vi "timeout determiner.vi"(11 "Status":T1={"VI"={"error"={"status"=FALSE, "code"=0, "source"=""}, "isExiting?"=FALSE}, "UserLoggedIn?"=FALSE, "AVI Refnum"=refnum, "video path"=path "", "Frame Data"={"Width"=0, "Height"=0, "Frames Per Second"=0, "Codec"="", "Has Data"=FALSE}, "Number of Frames"=0, "Frame Number"=0, "Image Placeholder"=refnum, "Image Output"=refnum, "First Frame?"=TRUE, "Running?"=FALSE, "ROI Type"=enum."Line ROI", "ROI Descriptor"={"Global Rectangle"=[], "Contours"=[]}, "ROI Present?"=FALSE, "Filter Set?"=FALSE, "Loop?"=FALSE, "Filtering?"=FALSE, "Filter Parameters"={"Sigma"=1.0, "HThresh"=0.7, "LThres"=0.2, "WindowSize"=9}} {"Filter Parameters"."LThres" min=0 max=1 format="%.2f"; "Filter Parameters"."HThresh" min=0 max=1 format="%.2f"; "Filter Parameters"."Sigma" min=0 max=1 format="%.2f"; "ROI Descriptor"."Contours"."Type" items=["No Selection", "Point", "Line", "Rectangle", "Oval", "Polygon", "Freehand Region", "Annulus", "Unused2", "Unused3", "Broken Line", "Freehand Line", "Rotated Rectangle"]}) -> (3 "Numeric":i32)   [LabVIEW 2018]
uses:
  Status.ctl
  <vilib>/vision/Avi.llb/IMAQ AVI2 Refnum.ctl
  <vilib>/vision/Image Controls.llb/IMAQ Image.ctl
  ROI STYP.ctl
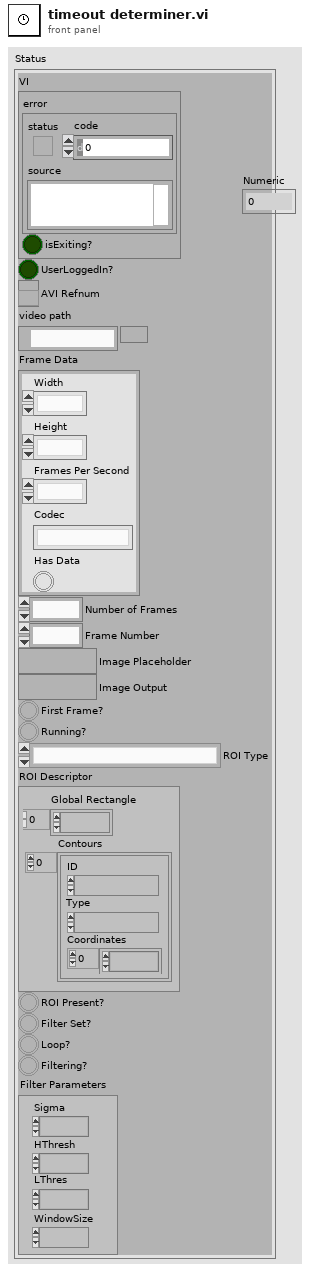
[diagram p1: front panel]
types:
  T1 = typedef "Status.ctl" = cluster{"VI":cluster{"error":errorcluster, "isExiting?":bool}, "UserLoggedIn?":bool, "AVI Refnum":T2, "video path":path, "Frame Data":cluster{"Width":u32, "Height":u32, "Frames Per Second":u32, "Codec":string, "Has Data":bool}, "Number of Frames":i32, "Frame Number":u32, "Image Placeholder":T3, "Image Output":T3, "First Frame?":bool, "Running?":bool, "ROI Type":T4, "ROI Descriptor":T5, "ROI Present?":bool, "Filter Set?":bool, "Loop?":bool, "Filtering?":bool, "Filter Parameters":cluster{"Sigma":sgl, "HThresh":sgl, "LThres":sgl, "WindowSize":i32}}
  T2 = typedef "IMAQ AVI2 Refnum.ctl" = refnum<k20>
  T3 = typedef "IMAQ Image.ctl" = refnum<image>
  T4 = typedef "ROI STYP.ctl" = enum16{"Line ROI", "Rectangle ROI", "Freeform ROI"}
  T5 = typedef "ROI Descriptor" = cluster{"Global Rectangle":i32[], "Contours":cluster{"ID":enum32{"External", "Internal"}, "Type":u32, "Coordinates":i32[]}[]}
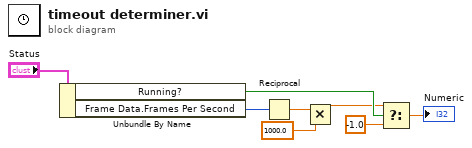
[diagram p0: block diagram]
diagram:
  n1 = Unbundle By Name("Status") -> ("Running?"=w3:bool, "Frame Data.Frames Per Second"=w7:u32)
  n2 = Reciprocal(x=w7) -> (1/x=w6:dbl)
  n3 = Multiply(x=w6, y=1000.0) -> (x*y=w2:dbl)
  n4 = Select(t=w2, s=w3, f=-1.0) -> (s? t:f=→"Numeric":dbl)
